vi "DSF.Engine.Sequencer.Get Plugin Timings.vi"(8 "error in (no error)":errorcluster, 11 "Sequencer in":refnum<class "DSF.Engine.Sequencer.lvclass">) -> (0 "error out":errorcluster, 2 "Plugin Timings":refnum<class "DSF.Engine.Timing.lvclass">[](array[class]), 3 "Sequencer out":refnum<class "DSF.Engine.Sequencer.lvclass">)   [LabVIEW 2016, in "DSF.Engine.lvlib" / "DSF.Engine.Sequencer.lvclass"]
uses:
  DSF.Engine.Sequencer.lvclass
  Timing/DSF.Engine.Timing.lvclass
  DSF.Engine.Sequencer.lvclass/DSF.Engine.Sequencer.ctl
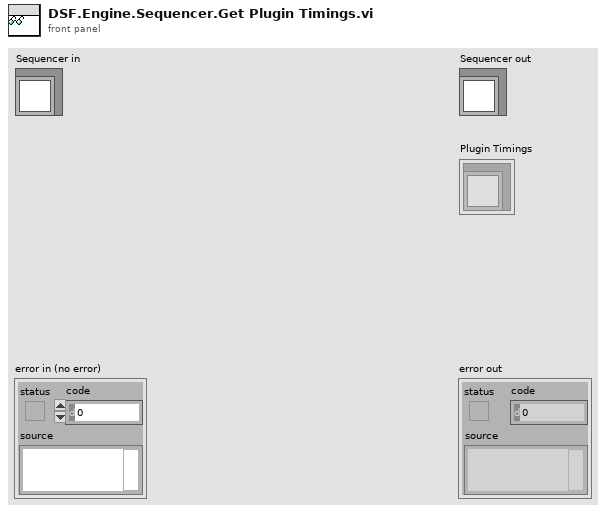
[diagram p1: front panel]
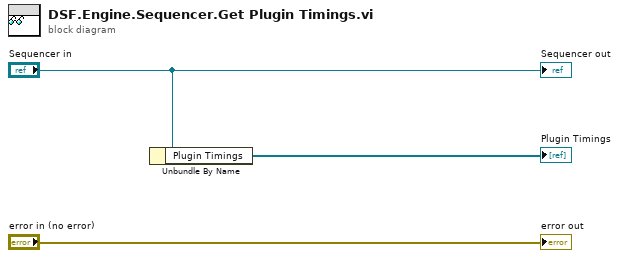
[diagram p0: block diagram]
diagram:
  n1 = Unbundle By Name("Sequencer in") -> ("Plugin Timings"=→"Plugin Timings":refnum<class "DSF.Engine.Timing.lvclass">[])
  "error out" <- "error in (no error)"
  "Sequencer out" <- "Sequencer in"
